vi "NonLinearAmp.vi"() -> ()   [LabVIEW 2009]
uses:
  <vilib>/measure/maspectr.llb/FFT Power Spectrum for 1 Chan.vi
  <vilib>/measure/NI_MAPro.lvlib
panel:
  in  "Tab Control":enum32{"Amplifier Input", "Amplifier Output"}(tab)=enum."Amplifier Output"
  out "Amplifier Input (Time Domain)":waveform(dbl)(graph)={"t0"=timestamp(0 s since 1904-01-01), "dt"=5.201831044527674e-11, "Y"=array[96120 elements]}
  out "Amplifier Input Spectrum (Frequency Domain - Magnitude)":cluster{"f0":dbl, "df":dbl, dbl[]}(graph)={"f0"=0.0, "df"=199999.99999999997, array[48060 elements]}
  out "Amplifier Output Spectrum (Frequency Domain - Magnitude)":cluster{"f0":dbl, "df":dbl, dbl[]}(graph)={"f0"=0.0, "df"=199999.99999999997, array[48060 elements]}
  out "Amplifier Output (Time Domain)":waveform(dbl)(graph)={"t0"=timestamp(0 s since 1904-01-01), "dt"=5.201831044527674e-11, "Y"=array[96120 elements]}
  in  "Amplifier Gain Terms (first gain term applied to linear part)":dbl[](array[numeric])=[10.0, 0.005, 0.0, 0.0, 0.0] format="%.2p"
  in  "Show Intermodulation Distortion":bool
  in  "Show Harmonic Distortion":bool=TRUE
  in  "Duration (seconds)":dbl=5e-06 min=0.0
  in  "Integer Degree of Nonlinearity":i32=2 caption="Integer Degree of Nonlinearity (N) ( y(t) = x^1(t) + ...  + x^N(t) )"
  in  "Tone Frequencies":dbl[](array[numeric])=[800000000.0, 801000000.0] format="%.2p"
  in  "Tone Power (dBm)":dbl[](array[numeric])=[0.0, -300.0] format="%.2p"
  # "Configuration"
  # "*For more information on each a control, please see the description for that control"
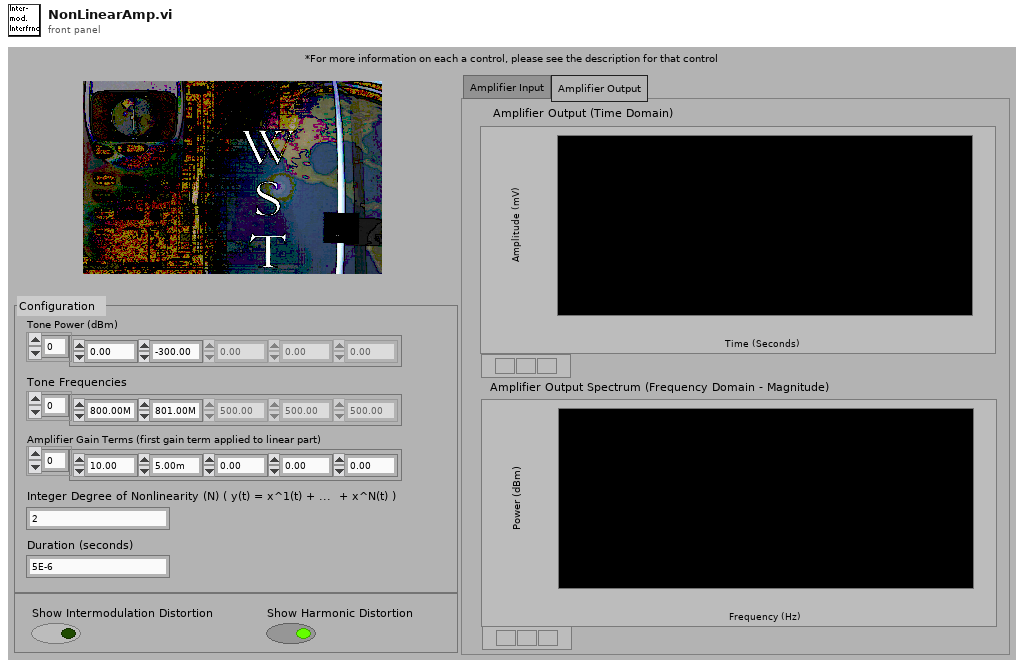
[diagram p1: front panel]
types:
  T1 = enum16{"None ", "Hanning", "Hamming", "Blackman-Harris", "Exact Blackman", "Blackman", "Flat Top", "4 Term B-Harris ", "7 Term B-Harris", "Low Sidelobe"}
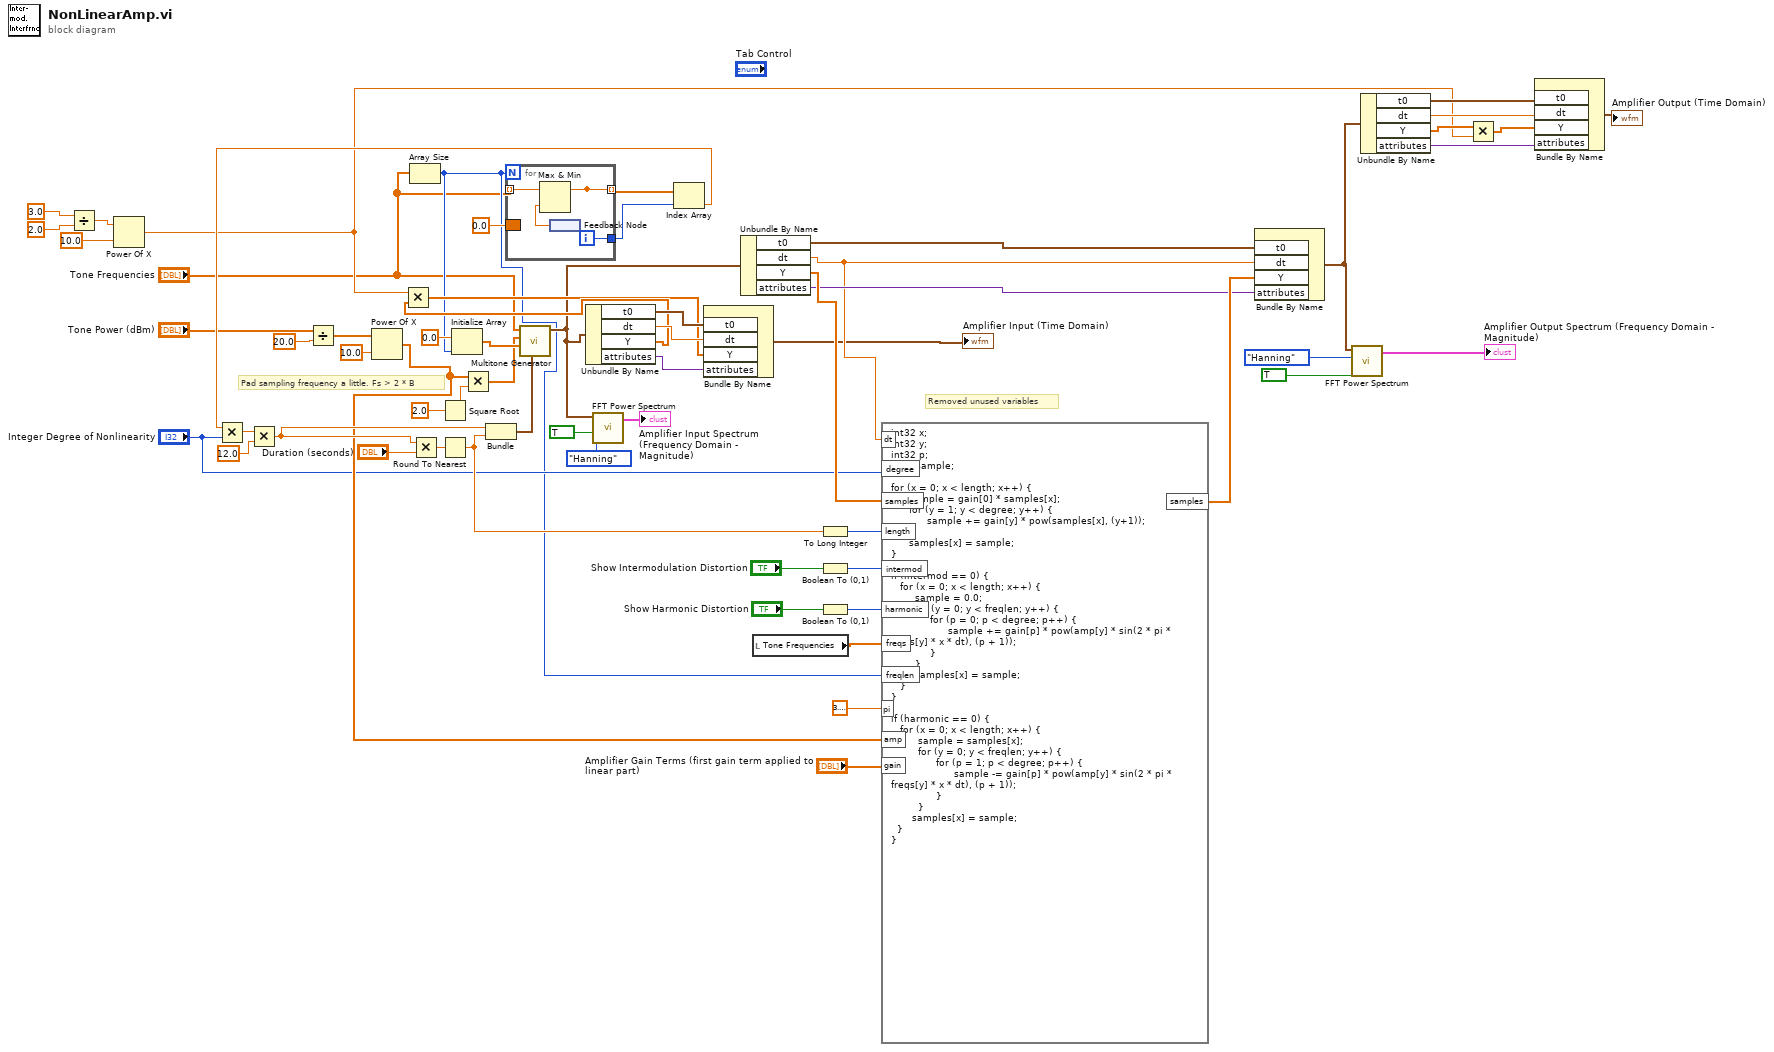
[diagram p0: block diagram]
diagram:
  # "Removed unused variables"
  # "Pad sampling frequency a little. Fs > 2 * B"
  n1 = Divide(x=3.0, y=2.0) -> (x/y=w28:dbl)
  n2 = Power Of X(1:10.0 ("x"), 2:w28) -> (0:w6:dbl)
  n3 = Divide(x="Tone Power (dBm)", y=20.0) -> (x/y=w32:dbl[])
  n4 = Power Of X(1:10.0 ("x"), 2:w32) -> (0:w8:dbl[])
  n5 = Array Size(array="Tone Frequencies") -> (size(s)=w4:i32)
  n6 = Square Root(x=2.0) -> (sqrt(x)=w11:dbl)
  n7 = Initialize Array(0.0 ("element"), w4) -> (w27:dbl[])
  n8 = Multiply(x=w8, y=w11) -> (x*y=w10:dbl[])
  n9 = for {
    N: w4 -> [_]
    tunnel: "Tone Frequencies" -> [w66] mode=indexing
    tunnel: [w64] -> w61 mode=indexing
    tunnel: [w63] -> w3
    border: 0.0 -> [_]
    i -> [w63]
    n10 = feedback #1() -> (w65:dbl)
    n11 = Max & Min(x=w66, y=w65) -> (max(x,y)=w64:dbl)  [unwired: 1 out]
  }
  n12 = Index Array(array=w61, index=w3) -> (element=w60:dbl)
  n13 = Multiply(x=w60, y="Integer Degree of Nonlinearity") -> (x*y=w50:dbl)
  n14 = Multiply(x=w50, y=12.0) -> (x*y=w38:dbl)
  n15 = Multiply(x=w38, y="Duration (seconds)") -> (x*y=w48:dbl)
  n16 = Round To Nearest(number=w48) -> (nearest integer value=w47:dbl)
  n17 = Bundle(w38, w47) -> (w26:cluster{dbl, dbl})  [unwired: 1 in]
  n18 = call <vilib>:"Multitone Generator.vi"("sampling info"=w26, "tone phases"=w27, "tone amplitudes"=w10, "tone frequencies"="Tone Frequencies") -> ("signal out"=w13:waveform(dbl))  [unwired: 4 in, 3 out]
  n19 = Unbundle By Name(w13) -> ("t0"=w21:timestamp, "dt"=w22:dbl, "Y"=w20:dbl[], "attributes"=w23:variant)
  n20 = Multiply(x=w6, y=w20) -> (x*y=w19:dbl[])
  n21 = call-poly <vilib>:"FFT Power Spectrum.vi"("dB On (F)"=TRUE, "window"=T1."Hanning", "time signal"=w13) -> ("power spectrum"=→"Amplifier Input Spectrum (Frequency Domain - Magnitude)":cluster{"f0":dbl, "df":dbl, "magnitude":dbl[]})  [unwired: 5 in, 3 out]
  n22 = Bundle By Name("t0"=w21, "dt"=w22, "Y"=w19, "attributes"=w23) -> (→"Amplifier Input (Time Domain)":waveform(dbl))  [unwired: 1 in]
  n23 = Unbundle By Name(w13) -> ("t0"=w51:timestamp, "dt"=w46:dbl, "Y"=w59:dbl[], "attributes"=w52:variant)
  n24 = local read "Tone Frequencies"() -> (w1:dbl[])
  n25 = To Long Integer(number=w47) -> (32bit integer=w58:i32)
  n26 = Boolean To (0,1)(Boolean="Show Intermodulation Distortion") -> (0, 1=w57:i16)
  n27 = Boolean To (0,1)(Boolean="Show Harmonic Distortion") -> (0, 1=w56:i16)
  n28 = formula code="int32 x;\nint32 y;\nint32 p;\nfloat sample;\n\nfor (x = 0; x < length; x++) {\n      sample = gain[0] * samples[x];\n      for (y = 1; y < degree; y++) {\n            sample += gain[y] * pow(samples[x], (y+1));  \n      }\n      samples[x] = sample;\n}\n\nif (intermod == 0) {\n   for (x = 0; x < length; x++) {\n        sample = 0.0;\n        for (y = 0; y < freqlen; y++) {\n             for (p = 0; p < degree; p++) {\n                   sample += gain[p] * pow(amp[y] * sin(2 * pi * freqs[y] * x * dt), (p + 1));\n             }\n        }\n        samples[x] = sample;\n   }\n}\n\nif (harmonic == 0) {\n   for (x = 0; x < length; x++) {\n         sample = samples[x];\n         for (y = 0; y < freqlen; y++) {\n               for (p = 1; p < degree; p++) {\n                     sample -= gain[p] * pow(amp[y] * sin(2 * pi * freqs[y] * x * dt), (p + 1));\n               }\n         }\n       samples[x] = sample;\n  }\n}"("degree"="Integer Degree of Nonlinearity", "samples"=w59, "length"=w58, "intermod"=w57, "harmonic"=w56, "dt"=w46, "freqs"=w1, "freqlen"=w4, "pi"=3.141592653589793, "amp"=w8, "gain"="Amplifier Gain Terms (first gain term applied to linear part)") -> ("samples"=w53:dbl[])
  n29 = Bundle By Name("t0"=w51, "dt"=w46, "Y"=w53, "attributes"=w52) -> (w25:waveform(dbl))  [unwired: 1 in]
  n30 = call-poly <vilib>:"FFT Power Spectrum.vi"("dB On (F)"=TRUE, "window"=T1."Hanning", "time signal"=w25) -> ("power spectrum"=→"Amplifier Output Spectrum (Frequency Domain - Magnitude)":cluster{"f0":dbl, "df":dbl, "magnitude":dbl[]})  [unwired: 5 in, 3 out]
  n31 = Unbundle By Name(w25) -> ("t0"=w18:timestamp, "dt"=w17:dbl, "Y"=w15:dbl[], "attributes"=w16:variant)
  n32 = Multiply(x=w15, y=w6) -> (x*y=w14:dbl[])
  n33 = Bundle By Name("t0"=w18, "dt"=w17, "Y"=w14, "attributes"=w16) -> (→"Amplifier Output (Time Domain)":waveform(dbl))  [unwired: 1 in]
